vi "Convert matlab to TDMS data.vi"() -> ()   [LabVIEW 2014]
uses:
  <vilib>/Platform/storage/lvStorage.llb/_openFunction.ctl
  <vilib>/Platform/storage/lvStorage.llb/_openStorageWithRootAutoDetect.vi
  <vilib>/Platform/storage/lvStorage.llb/xStorage/xStorageSupp/ErrorOut.vi
  <vilib>/Platform/storage/lvStorage.llb/_queryPropPoly.vi
  <vilib>/Platform/storage/lvStorage.llb/_queryPropString.vi
  <vilib>/Platform/storage/lvStorage.llb/_queryGenericObjects.vi
  <vilib>/Platform/storage/lvStorage.llb/_loadAllDdt.vi
  <vilib>/Platform/storage/Storage.llb/Get Object Info.vi
  <vilib>/Platform/storage/Storage.llb/__closeStorageFromObject.vi
  <vilib>/Platform/storage/lvStorage.llb/xStorage/Open Data Storage/Open Data Storage.xnode
  <vilib>/Platform/storage/lvStorage.llb/xStorage/Read Data/Read Data.xnode
  <vilib>/Platform/storage/lvStorage.llb/xStorage/Close Data Storage/Close Data Storage.xnode
panel:
  in  "Input File":path
  in  "Output File":path
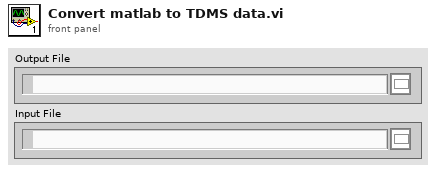
[diagram p1: front panel]
types:
  T1 = enum16{"open", "open or create", "create or replace", "create", "open (read-only)"}
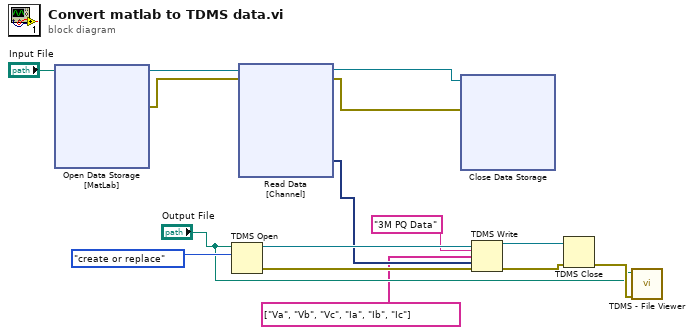
[diagram p0: block diagram]
diagram:
  n1 = xnode "Open Data Storage\n[MatLab]"("file path"="Input File") -> ("storage refnum (file)"=w15:refnum<k20>, "error out"=w12:errorcluster)  [unwired: 4 in, 1 out]
  n2 = TDMS Open(10:T1."create or replace" ("operation (0:open)"), 11:"Output File") -> (0:w8:errorcluster, 3:w9:refnum<k34>)  [unwired: 5 in]
  n3 = xnode "Read Data\n[Channel]"("storage refnum (file)"=w15, "error in"=w12) -> ("Signal"=w7:dynamicdata, "storage refnum (file) out"=w14:refnum<k20>, "error out"=w13:errorcluster)  [unwired: 2 in, 1 out]
  n4 = xnode "Close Data Storage\n"("storage refnum (file)"=w14, "error in (no error)"=w13) -> ()  [unwired: 2 out]
  n5 = TDMS Write(0:w9, 5:"3M PQ Data" ("group name in (Untitled)"), 7:string[] ["Va", "Vb", "Vc", "Ia", "Ib", "Ic"] ("channel name(s) in (Untitled)"), 9:w7, 11:w8) -> (4:w6:refnum<k34>, 15:w5:errorcluster)  [unwired: 1 in, 2 out]
  n6 = TDMS Close(8:w5, 11:w6) -> (0:w4:errorcluster)  [unwired: 1 out]
  n7 = call <vilib>:"TDMS - File Viewer.vi"("error in (no error)"=w4, "file path"="Output File") -> ()  [unwired: 4 in, 2 out]
